vi "pathtest.vi"() -> ()   [LabVIEW 2012]
panel:
  out "appended path":path
  in  "Msg Package Path (blank)":path
  in  "Message Type":string
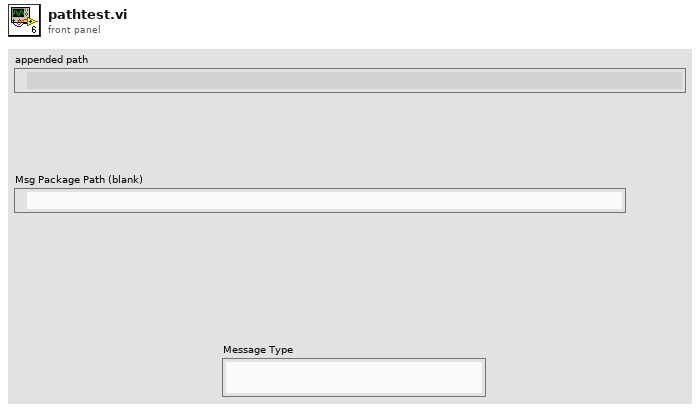
[diagram p1: front panel]
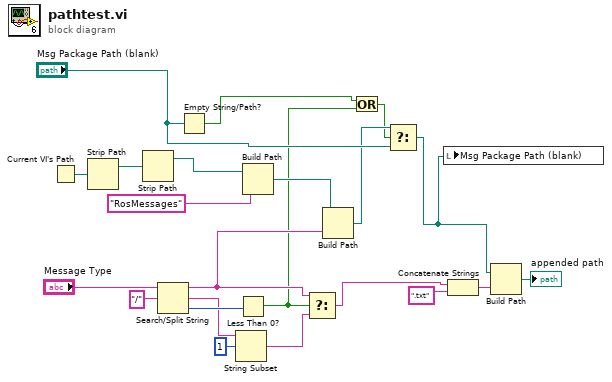
[diagram p0: block diagram]
diagram:
  n1 = Current VI's Path() -> (path=w22:path)
  n2 = Strip Path(path=w22) -> (stripped path=w21:path)  [unwired: 1 out]
  n3 = Strip Path(path=w21) -> (stripped path=w20:path)  [unwired: 1 out]
  n4 = Search/Split String(string="Message Type", search string/char (-)="/") -> (substring before match=w11:string, match + rest of string=w8:string, offset of match=w12:i32)  [unwired: 1 in]
  n5 = Empty String/Path?(string/path="Msg Package Path (blank)") -> (empty?=w5:bool)
  n6 = String Subset(string=w8, offset (0)=1) -> (substring=w6:string)  [unwired: 1 in]
  n7 = Less Than 0?(x=w12) -> (x < 0?=w1:bool)
  n8 = Build Path(base path=w20, name or relative path="RosMessages") -> (appended path=w16:path)
  n9 = Select(t=w11, s=w1, f=w6) -> (s? t:f=w10:string)
  n10 = Build Path(base path=w16, name or relative path=w11) -> (appended path=w3:path)
  n11 = Or(x=w5, y=w1) -> (x .or. y?=w2:bool)
  n12 = Select(t=w3, s=w2, f="Msg Package Path (blank)") -> (s? t:f=w13:path)
  n13 = local write "Msg Package Path (blank)"(w13) -> ()
  n14 = Concatenate Strings(w10, ".txt" ("string")) -> (w15:string)
  n15 = Build Path(base path=w13, name or relative path=w15) -> (appended path=→"appended path":path)
